vi "Real FFT PtByPt.vi"(2 "initialize":bool, 3 "sample length":i32=100, 5 "x":dbl format="%0.2f") -> (0 "error":i32, 1 "FFT{X}":cdb[](array[numeric]))   [LabVIEW 2020, in "NI_PtbyPt.lvlib"]
doc: "Computes the Fourier transform of <B>x</B>. This VI is similar to the FFT VI. Wire data to the <B>x</B> input to determine the polymorphic instance to use or manually select the instance."
uses:
  <vilib>/ptbypt/NI_PtbyPt.lvlib
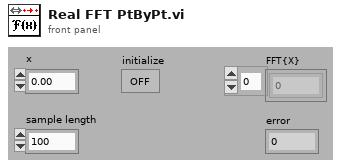
[diagram p1: front panel]
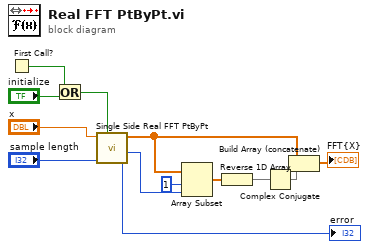
[diagram p0: block diagram]
diagram:
  n1 = First Call?() -> (First Call?: T/F=w1:bool)
  n2 = Or(x=w1, y="initialize") -> (x .or. y?=w2:bool)
  n3 = call <vilib>:"Single Side Real FFT PtByPt.vi"("initialize"=w2, "sample length"="sample length", "input data"="x") -> ("error"=→"error":i32, "half length"=w7:i32, "FFT Single Side"=w6:cdb[])  [unwired: 2 in, 1 out]
  n4 = Array Subset(array=w6, index=1 ("Array Index"), length=w7) -> (w11:cdb[])
  n5 = Reverse 1D Array(array=w11) -> (reversed array=w10:cdb[])
  n6 = Complex Conjugate(1:w10) -> (0:w9:cdb[])
  n7 = Build Array (concatenate)(w6, w9) -> (→"FFT{X}":cdb[])
